vi "UTILITY Boolean Queue.vi"(7 "Status":T1, 8 "error in (no error)":errorcluster, 10 "Set Status":bool, 11 "name (unnamed)":string) -> (0 "error out":errorcluster, 2 "# elements in queue":i32, 3 "latest READ notification":bool)   [LabVIEW 2014]
uses:
  Type Definitions/UTILITY Notifier.ctl
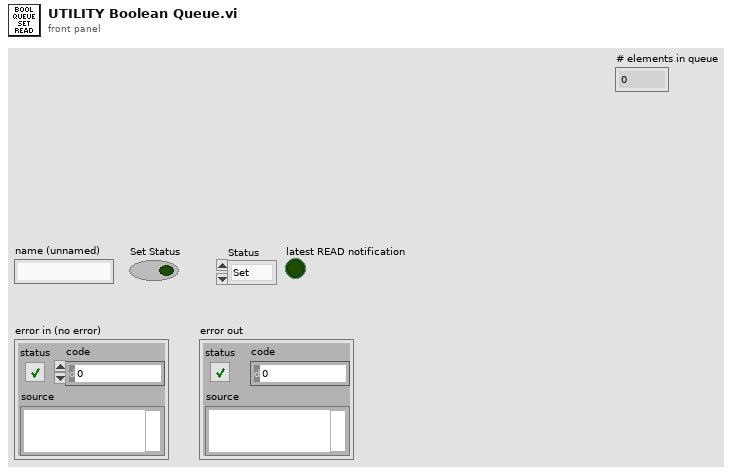
[diagram p1: front panel]
types:
  T1 = typedef "UTILITY Notifier.ctl" = enum16{"Set", "Read", "Release Ref"}
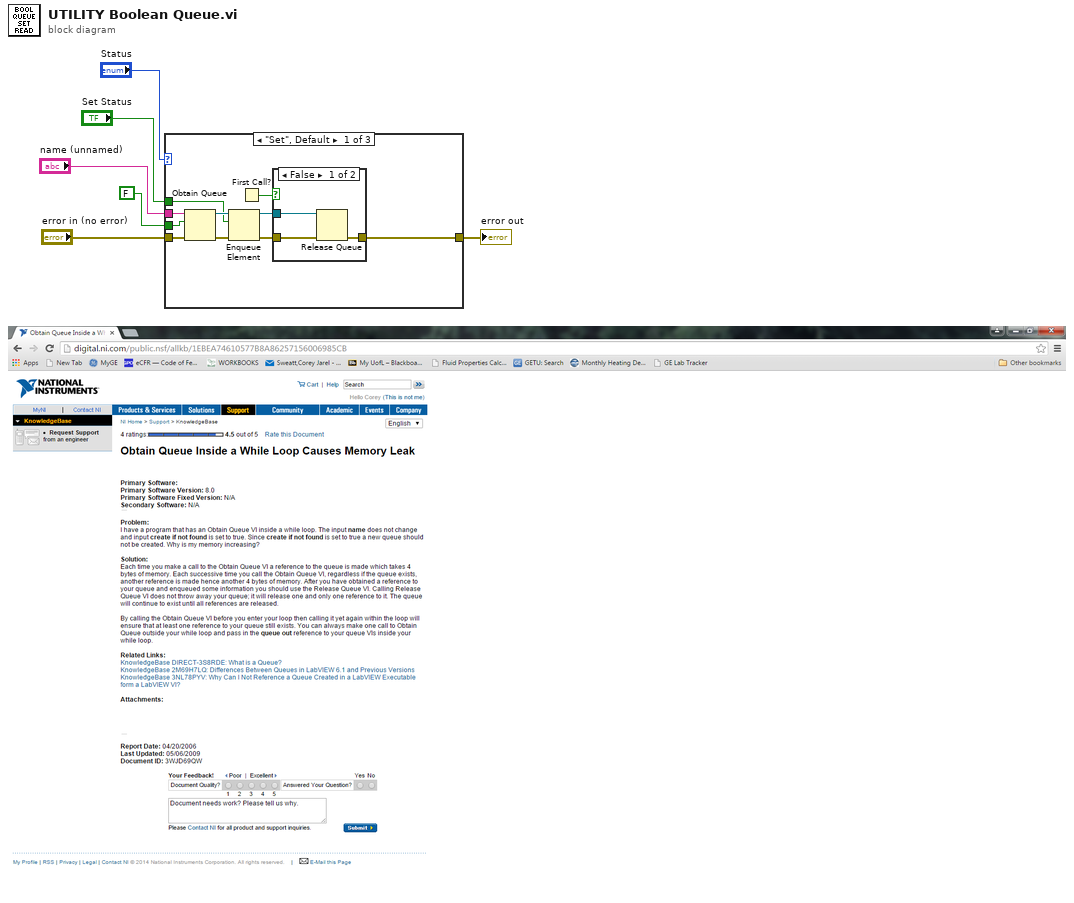
[diagram p0: block diagram]
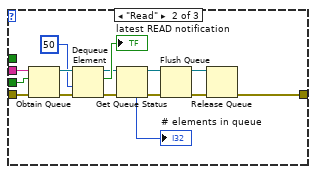
[diagram p3: hidden frame]
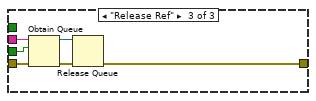
[diagram p4: hidden frame]
diagram:
  n1 = case shown="\"Set\", Default" "Status" {
    tunnel: [w9 w21 w37] -> w6
    tunnel: "error in (no error)" -> [w14 w33 w36]
    tunnel: "name (unnamed)" -> [w13 w31 w41]
    tunnel: "Set Status" -> [w12 _ _]
    tunnel: FALSE ("Aisle 1 Update") -> [w11 w30 w40]
    frame "Set", Default {
      n2 = Obtain Queue(name (unnamed)=w13, element data type=w11, error in (no error)=w14) -> (queue out=w15:refnum<queue>, error out=w16:errorcluster)  [unwired: 2 in, 1 out]
      n3 = Enqueue Element(queue=w15, element=w12, error in (no error)=w16) -> (queue out=w7:refnum<queue>, error out=w10:errorcluster)  [unwired: 1 in, 1 out]
      n4 = First Call?() -> (First Call?: T/F=w8:bool)
      n5 = case shown="False" w8 {
        tunnel: w10 -> [w19 w20]
        tunnel: [w18 w20] -> w9
        tunnel: w7 -> [w17 _]
        frame False {
          n6 = Release Queue(queue=w17, error in (no error)=w19) -> (error out=w18:errorcluster)  [unwired: 1 in, 2 out]
        }
        frame True {
        }
      }
    }
    frame "Read" {
      n7 = Obtain Queue(name (unnamed)=w31, element data type=w30, error in (no error)=w33) -> (queue out=w34:refnum<queue>, error out=w35:errorcluster)  [unwired: 2 in, 1 out]
      n8 = Dequeue Element(queue=w34, timeout in ms (-1)=50, error in (no error)=w35) -> (queue out=w28:refnum<queue>, element=→"latest READ notification":bool, error out=w29:errorcluster)  [unwired: 1 out]
      n9 = Get Queue Status(queue=w28, error in (no error)=w29) -> (queue out=w24:refnum<queue>, error out=w25:errorcluster, # elements in queue=→"# elements in queue":i32)  [unwired: 1 in, 5 out]
      n10 = Flush Queue(queue=w24, error in (no error)=w25) -> (queue out=w23:refnum<queue>, error out=w22:errorcluster)  [unwired: 1 out]
      n11 = Release Queue(queue=w23, error in (no error)=w22) -> (error out=w21:errorcluster)  [unwired: 1 in, 2 out]
    }
    frame "Release Ref" {
      n12 = Obtain Queue(name (unnamed)=w41, element data type=w40, error in (no error)=w36) -> (queue out=w39:refnum<queue>, error out=w38:errorcluster)  [unwired: 2 in, 1 out]
      n13 = Release Queue(queue=w39, error in (no error)=w38) -> (error out=w37:errorcluster)  [unwired: 1 in, 2 out]
    }
  }
  "error out" <- w6
